vi "Loop (Data Stream).vi"(8 "Error IN":errorcluster) -> (0 "Error OUT":errorcluster)   [LabVIEW 2013]
uses:
  Real-Time/Controls/TCP Data Stream Mode (RT).ctl
  Real-Time/Controls/RT FIFO Mode.ctl
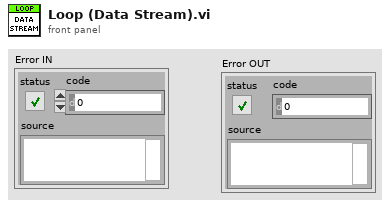
[diagram p1: front panel]
types:
  T1 = typedef "TCP Data Stream Mode (RT).ctl" = enum16{"Init", "Write Data", "Close"}
  T2 = typedef "RT FIFO Mode.ctl" = enum16{"Create", "Write", "Read", "Delete"}
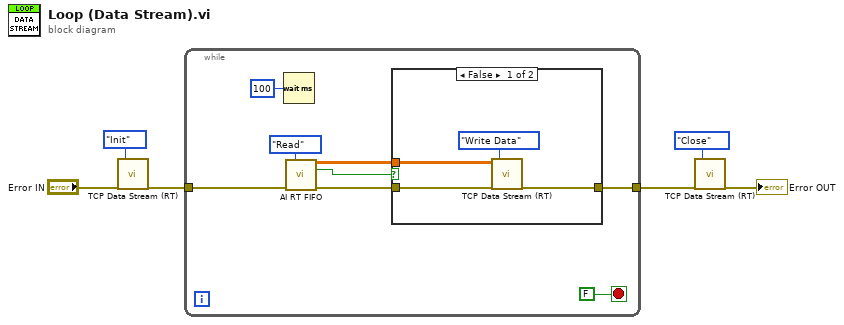
[diagram p0: block diagram]
diagram:
  n1 = call "TCP Data Stream (RT).vi"("Error IN"="Error IN", "Mode"=TCP_Data_Stream_Mode_(RT)."Init") -> ("Error OUT"=w6:errorcluster)  [unwired: 16 in, 1 out]
  n2 = while {
    tunnel: w6 -> [w14]
    tunnel: [w12] -> w2
    stop <- FALSE stop-if-true
    n3 = Wait (ms)(milliseconds to wait=u32 100) -> ()  [unwired: 1 out]
    n4 = call "AI RT FIFO.vi"("Mode"=RT_FIFO_Mode."Read", "Error IN"=w14) -> ("Data OUT"=w10:dbl[][], "Empty?"=w13:bool, "Error OUT"=w11:errorcluster)  [unwired: 11 in]
    n5 = case shown="False" w13 {
      tunnel: w10 -> [w17 _]
      tunnel: [w15 w19] -> w12
      tunnel: w11 -> [w16 w19]
      frame False {
        n6 = call "TCP Data Stream (RT).vi"("Data"=w17, "Error IN"=w16, "Mode"=TCP_Data_Stream_Mode_(RT)."Write Data") -> ("Error OUT"=w15:errorcluster)  [unwired: 15 in, 1 out]
      }
      frame True {
      }
    }
  }
  n7 = call "TCP Data Stream (RT).vi"("Error IN"=w2, "Mode"=TCP_Data_Stream_Mode_(RT)."Close") -> ("Error OUT"=→"Error OUT":errorcluster)  [unwired: 16 in, 1 out]
